vi "Result.Parse Data File Name to SN, Time, Result.vi"(11 "File Path":path) -> (0 "CT Image File Path":path, 1 "DateTime":timestamp, 2 "SN":string, 3 "Pass":bool, 4 "ImageName":string)   [LabVIEW 2019]
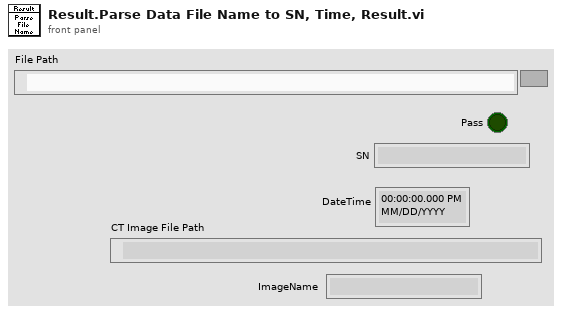
[diagram p1: front panel]
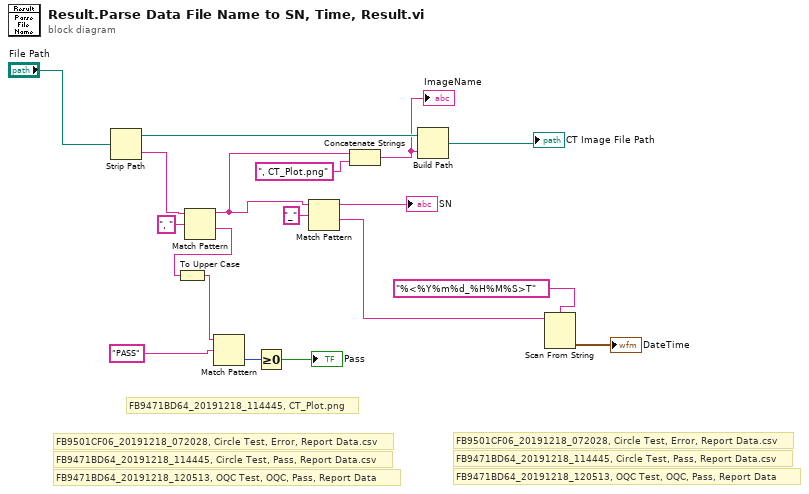
[diagram p0: block diagram]
diagram:
  # "FB9471BD64_20191218_120513, OQC Test, OQC, Pass, Report Data"
  # "FB9471BD64_20191218_114445, Circle Test, Pass, Report Data.csv"
  # "FB9501CF06_20191218_072028, Circle Test, Error, Report Data.csv"
  # "FB9471BD64_20191218_114445, CT_Plot.png"
  # "FB9471BD64_20191218_120513, OQC Test, OQC, Pass, Report Data"
  # "FB9471BD64_20191218_114445, Circle Test, Pass, Report Data.csv"
  # "FB9501CF06_20191218_072028, Circle Test, Error, Report Data.csv"
  n1 = Strip Path(path="File Path") -> (stripped path=w10:path, name=w16:string)
  n2 = Match Pattern(string=w16, regular expression=", ") -> (before substring=w6:string, after substring=w15:string)  [unwired: 1 in, 2 out]
  n3 = To Upper Case(1:w15) -> (0:w14:string)
  n4 = Match Pattern(string=w14, regular expression="PASS") -> (offset past match=w12:i32)  [unwired: 1 in, 3 out]
  n5 = Greater Or Equal To 0?(x=w12) -> (x >= 0?=→"Pass":bool)
  n6 = Match Pattern(string=w6, regular expression="_") -> (before substring=→"SN":string, after substring=w3:string)  [unwired: 1 in, 2 out]
  n7 = Concatenate Strings(w6, ", CT_Plot.png") -> (w1:string)
  "ImageName" <- w1
  n8 = Build Path(base path=w10, name or relative path=w1) -> (appended path=→"CT Image File Path":path)
  n9 = Scan From String(format string="%<%Y%m%d_%H%M%S>T", input string=w3) -> (output 1=→"DateTime":timestamp)  [unwired: 3 in, 3 out]
